vi "Read Main Stop Event .vi"(8 "error in (no error)":errorcluster, 11 "HGF_Application in":refnum<class "HGF_Application.lvclass">) -> (0 "error out":errorcluster, 2 "Main Stop Event":refnum<user-event>, 3 "HGF_Application out":refnum<class "HGF_Application.lvclass">)   [LabVIEW 2009]
uses:
  HGF_Application.lvclass
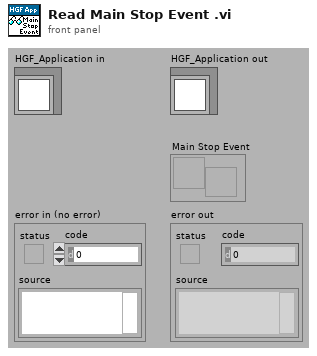
[diagram p1: front panel]
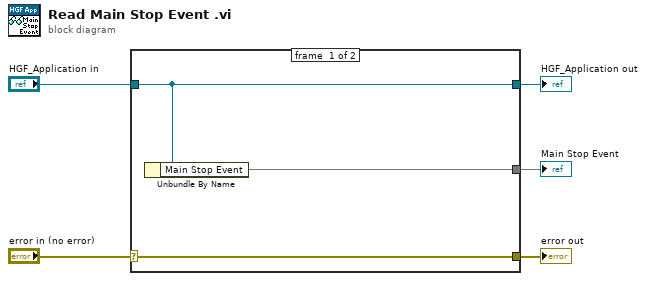
[diagram p0: block diagram]
diagram:
  n1 = case shown="No Error" "error in (no error)" {
    selector: "error in (no error)" -> [w8 w9]
    tunnel: [w8 w9] -> w4
    tunnel: [w7 w10] -> w2
    tunnel: "HGF_Application in" -> [w7 w10]
    tunnel: [w6 _] -> w1
    frame #0 {
      n2 = Unbundle By Name(w7) -> ("Main Stop Event"=w6)
    }
    frame #1 {
    }
  }
  "error out" <- w4
  "HGF_Application out" <- w2
  "Main Stop Event" <- w1
